vi "Parse URL.vi"(10 "Full":bool, 11 "URL":string="http://roborio-419-frc.local:1181/video?name=Camera&resolution=640x480&compression=40&fps=15") -> (0 "cgi string":string, 1 "parameters":T1(array[cluster]), 2 "port":i32, 3 "address":string)   [LabVIEW 2016]
panel:
  out "Array":T2(array[cluster])
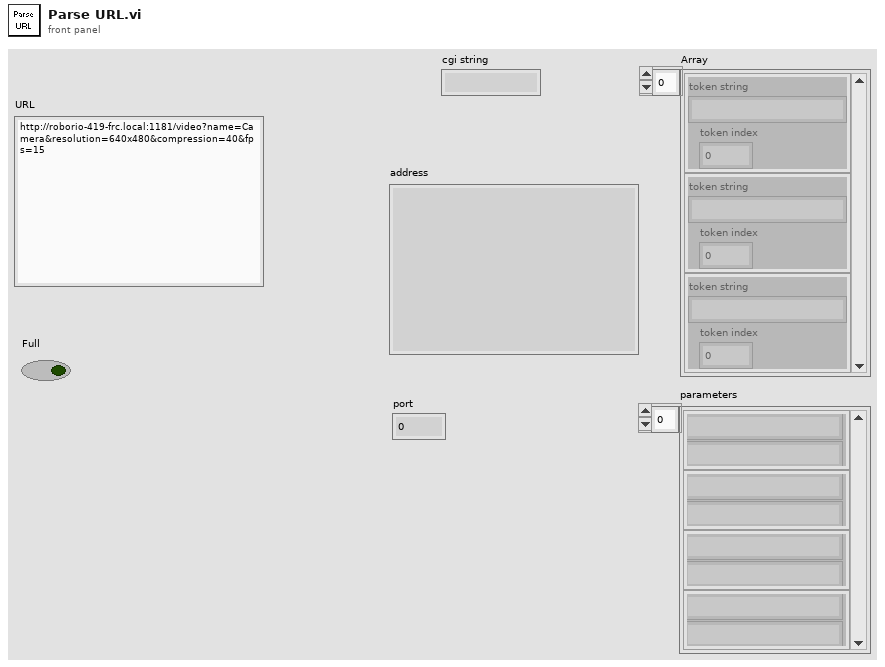
[diagram p1: front panel]
types:
  T1 = cluster{"token string":string, "token string 2":string}[]
  T2 = cluster{"token string":string, "token index":i32}[]
  T3 = cluster{"token string":string, "offset past token":i32}
  T4 = cluster{"token string":string, "offset past token":i32}[]
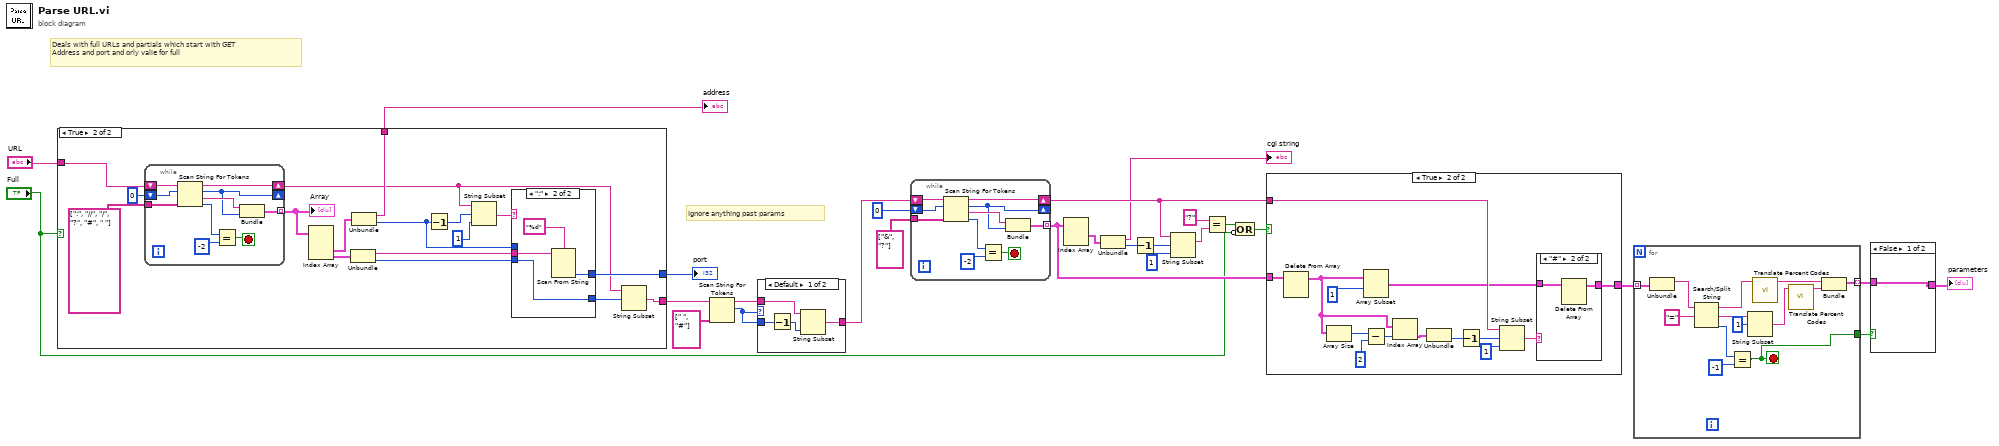
[diagram p0: block diagram]
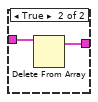
[diagram p3: hidden frame]
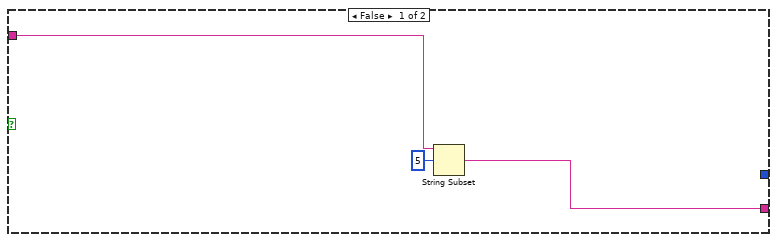
[diagram p4: hidden frame]
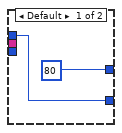
[diagram p5: hidden frame]
diagram:
  # "Ignore anything past params"
  # "Deals with full URLs and partials which start with GET \nAddress and port and orly valie for full"
  n1 = case shown="True" "Full" {
    tunnel: [_ w41] -> w26
    tunnel: [_ w40] -> w25
    tunnel: "URL" -> [w29 w36]
    tunnel: [w28 w35] -> w5
    frame False {
      n2 = String Subset(string=w29, offset (0)=5) -> (substring=w28:string)  [unwired: 1 in]
    }
    frame True {
      n3 = while {
        tunnel: string[] [":", "//", "/", "?", "#", " "] -> [w62]
        shift-right: [w60] -> w37
        shift-left: w36 -> [w61]
        shift-right: [w53] -> _
        shift-left: 0 ("offset past token") -> [w59]
        tunnel: [w54] -> w44 mode=indexing
        stop <- w57 stop-if-true
        n4 = Scan String For Tokens(6:w62, 8:w59, 9:w61) -> (0:w55:i32, 1:w56:string, 2:w53:i32, 3:w60:string)  [unwired: 3 in]
        n5 = Equal?(x=w55, y=-2) -> (x = y?=w57:bool)
        n6 = Bundle("token string"=w56, "offset past token"=w53) -> (w54:T3)  [unwired: 1 in]
      }
      "Array" <- w44
      n7 = Index Array(array=w44) -> (element #2=w43:T3, element #3=w42:T3)  [unwired: 3 in, 1 out]
      n8 = Unbundle(w42) -> ("token string"=w34:string, "offset past token"=w39:i32)
      n9 = Unbundle(w43) -> ("token string"=w40:string, "offset past token"=w38:i32)
      n10 = Decrement(x=w38) -> (x-1=w32:i32)
      n11 = String Subset(string=w37, offset (0)=w32, length (rest)=1) -> (substring=w31:string)
      n12 = case shown="\":\"" w31 {
        tunnel: w34 -> [_ w52]
        tunnel: [80 w50] -> w41
        tunnel: w39 -> [_ w49]
        tunnel: [w47 w49] -> w30
        tunnel: w38 -> [w47 _]
        frame Default {
        }
        frame ":" {
          n13 = Scan From String(format string="%d", input string=w52) -> (output 1=w50:i32)  [unwired: 3 in, 3 out]
        }
      }
      n14 = String Subset(string=w37, offset (0)=w30) -> (substring=w35:string)  [unwired: 1 in]
    }
  }
  "address" <- w25
  "port" <- w26
  n15 = Scan String For Tokens(6:string[] [" ", "#"], 9:w5) -> (2:w1:i32, 3:w2:string)  [unwired: 4 in, 2 out]
  n16 = case shown="Default" w1 {
    tunnel: w1 -> [w64 _]
    tunnel: [w65 w67] -> w3
    tunnel: w2 -> [w66 w67]
    frame Default {
      n17 = Decrement(x=w64) -> (x-1=w63:i32)
      n18 = String Subset(string=w66, length (rest)=w63) -> (substring=w65:string)  [unwired: 1 in]
    }
    frame -2, -1 {
    }
  }
  n19 = while {
    tunnel: string[] ["&", "?"] -> [w77]
    shift-right: [w75] -> w18
    shift-left: w3 -> [w76]
    shift-right: [w68] -> _
    shift-left: 0 ("offset past token") -> [w74]
    tunnel: [w69] -> w19 mode=indexing
    stop <- w72 stop-if-true
    n20 = Scan String For Tokens(6:w77, 8:w74, 9:w76) -> (0:w70:i32, 1:w71:string, 2:w68:i32, 3:w75:string)  [unwired: 3 in]
    n21 = Equal?(x=w70, y=-2) -> (x = y?=w72:bool)
    n22 = Bundle("token string"=w71, "offset past token"=w68) -> (w69:T3)  [unwired: 1 in]
  }
  n23 = Index Array(array=w19) -> (element #1=w16:T3)  [unwired: 2 in, 1 out]
  n24 = Unbundle(w16) -> ("token string"=→"cgi string":string, "offset past token"=w22:i32)
  n25 = Decrement(x=w22) -> (x-1=w21:i32)
  n26 = String Subset(string=w18, offset (0)=w21, length (rest)=1) -> (substring=w13:string)
  n27 = Equal?(x="?" ("format string"), y=w13) -> (x = y?=w12:bool)
  n28 = Compound Arithmetic op=OR(w12, invert "Full") -> (w11:bool)
  n29 = case shown="True" w11 {
    tunnel: w19 -> [_ w81]
    tunnel: w18 -> [_ w85]
    tunnel: [_ w82] -> w17
    frame False {
    }
    frame True {
      n30 = Delete From Array(array=w81) -> (array with subset deleted=w80:T4)  [unwired: 2 in, 1 out]
      n31 = Array Size(array=w80) -> (size(s)=w79:i32)
      n32 = Array Subset(array=w80, index=1) -> (w83:T4)  [unwired: 1 in]
      n33 = Subtract(x=w79, y=2) -> (x-y=w90:i32)
      n34 = Index Array(array=w80, index=w90) -> (element=w88:T3)
      n35 = Unbundle(w88) -> ("offset past token"=w89:i32)  [unwired: 1 out]
      n36 = Decrement(x=w89) -> (x-1=w86:i32)
      n37 = String Subset(string=w85, offset (0)=w86, length (rest)=1) -> (substring=w84:string)
      n38 = case shown="\"#\"" w84 {
        tunnel: w83 -> [w92 w94]
        tunnel: [w92 w93] -> w82
        frame "False", Default {
        }
        frame "#" {
          n39 = Delete From Array(array=w94) -> (array with subset deleted=w93:T4)  [unwired: 2 in, 1 out]
        }
      }
    }
  }
  n40 = for {
    tunnel: w17 -> [w107] mode=indexing
    tunnel: [w102] -> w7 mode=indexing
    tunnel: [w99] -> w8
    stop <- w99 stop-if-true
    n41 = Unbundle(w107) -> ("token string"=w103:string)  [unwired: 1 out]
    n42 = Search/Split String(string=w103, search string/char (-)="=" ("format string")) -> (substring before match=w98:string, match + rest of string=w105:string, offset of match=w100:i32)  [unwired: 1 in]
    n43 = Equal?(x=w100, y=-1 ("offset (0)")) -> (x = y?=w99:bool)
    n44 = String Subset(string=w105, offset (0)=1) -> (substring=w95:string)  [unwired: 1 in]
    n45 = call "Translate Percent Codes.vi"("String"=w98) -> ("String 2"=w97:string)  [unwired: 10 in]
    n46 = call "Translate Percent Codes.vi"("String"=w95) -> ("String 2"=w96:string)  [unwired: 10 in]
    n47 = Bundle("String 2"=w97, "String 2"=w96) -> (w102:cluster{"String 2":string, "String 2":string})  [unwired: 1 in]
  }
  n48 = case shown="False" w8 {
    tunnel: w7 -> [w108 w110]
    tunnel: [w108 w109] -> w6
    frame False {
    }
    frame True {
      n49 = Delete From Array(array=w110) -> (array with subset deleted=w109:cluster{"String 2":string, "String 2":string}[])  [unwired: 2 in, 1 out]
    }
  }
  "parameters" <- w6
